vi "UHR-Fleezers Control (host) -Leonardo 04-2018 V3_greenctrl.vi"(0 "Tab Green FB":T5(tab)=enum."Trap Control (RF)") -> ()   [LabVIEW 2013] (continued)
                  n1367 = call "isclickinwindow.vi"("Image Param"=w2127, "Point32"=w2126) -> ("Y px"=w2120:i32, "Height"=w2121:i32, "X px"=w2122:i32, "Width"=w2123:i32, "In image?"=w2125:bool)  [unwired: 1 in]
                  n1368 = Not(x=w2125) -> (.not. x?=w2124:bool)
                }
              }
            }
            n1369 = Not(x=w2078) -> (.not. x?=w2077:bool)
            n1370 = case shown="True" w2077 {
              tunnel: w2075 -> [_ w2141]
              tunnel: w2073 -> [_ w2140]
              tunnel: w2076 -> [_ w2139]
              tunnel: w2074 -> [_ w2138]
              frame False {
              }
              frame True {
                w2134 = FALSE ("Get Point")
                n1371 = local read "Scan lines (y)"() -> (w2143:u64)
                n1372 = local read "Actual MCL Inc (V)"() -> (w2135:dbl)
                n1373 = local read "Scan steps (MCL)"() -> (w2142:u64)
                n1374 = Divide "Y Pix/step"(x=w2138, y=w2143) -> (x/y=w2150:dbl)
                n1375 = Divide "Y V/pix"(x=w2135, y=w2150) -> (x/y=w2149:dbl)
                n1376 = Divide "Y half step offset"(x=w2135, y=2.0) -> (x/y=w2151:dbl)
                n1377 = Divide "X pix/step"(x=w2139, y=w2142) -> (x/y=w2148:dbl)
                n1378 = Negate(x=w2151) -> (-x=w2152:dbl)
                n1379 = local read "Initial Y"() -> (w2158:dbl)
                n1380 = Multiply(x=w2140, y=w2149) -> (x*y=w2159:dbl)
                n1381 = Divide "X half step offset"(x=w2135, y=2.0) -> (x/y=w2145:dbl)
                n1382 = Divide "X V/pix"(x=w2135, y=w2148) -> (x/y=w2147:dbl)
                n1383 = Multiply(x=w2135, y=w2142) -> (x*y=w2154:dbl)
                n1384 = Compound Arithmetic op=ADD(w2152, w2159, w2158) -> (w2136:dbl)
                "Pointer Y (V)" <- w2136
                n1385 = Multiply(x=w2147, y=w2141) -> (x*y=w2156:dbl)
                n1386 = Negate(x=w2145) -> (-x=w2144:dbl)
                n1387 = local read "Initial X"() -> (w2157:dbl)
                n1388 = Negate(x=w2156) -> (-x=w2155:dbl)
                n1389 = Compound Arithmetic op=ADD(w2144, w2154, w2157, w2155) -> (w2137:dbl)
                "Pointer X (V)" <- w2137
                n1390 = Or(x="Set X Only", y="Set Confocal Spot (X-Y)") -> (x .or. y?=w2130:bool)
                n1391 = Or(x="Set Confocal Spot (X-Y)", y="Set Y Only") -> (x .or. y?=w2129:bool)
                n1392 = case shown="True" w2130 {
                  tunnel: w2137 -> [_ w2160]
                  frame False {
                  }
                  frame True {
                    n1393 = property on="AO2" class="Slide (strict)"("Val(Sgnl)"=w2160) -> ()  [unwired: 2 in, 2 out]
                  }
                }
                n1394 = case shown="True" w2129 {
                  tunnel: w2136 -> [_ w2161]
                  frame False {
                  }
                  frame True {
                    n1395 = property on="AO1" class="Slide (strict)"("Val(Sgnl)"=w2161) -> ()  [unwired: 2 in, 2 out]
                  }
                }
                n1396 = local write "Set Confocal Spot (X-Y)"(w2134) -> ()
                n1397 = local write "Set X Only"(w2134) -> ()
                n1398 = local write "Set Y Only"(w2134) -> ()
              }
            }
          }
          frame 3 {
            n1399 = local read "BD 2 Frequency 1 (MHz)"() -> (w2162:dbl)
            n1400 = local read "BD 1 Frequency 1 (MHz)"() -> (w2163:dbl)
            n1401 = local write "Manipulating Trap"(TRUE ("Manipulating Trap")) -> ()
            n1402 = local write "Coords"(T8 {"Horizontal"=0, "Vertical"=0} ("Coords")) -> ()
            n1403 = while {
              tunnel: w2168 -> [w2173]
              tunnel: w2166 -> [w2172]
              tunnel: w2164 -> [w2171]
              tunnel: w2163 -> [w2170]
              tunnel: w2162 -> [w2169]
              stop <- w2174 stop-if-true
              n1404 = event shown="[0] \"Pane\": Mouse Move" {
                selector: _ -> [_ _]
                dyn-events: _ -> [_ _]
                timeout: _ -> [_ _]
                tunnel: ["Force Manip Abort" w2238] -> w2174
                tunnel: w2173 -> [w2181 _]
                tunnel: w2172 -> [w2179 _]
                tunnel: w2171 -> [w2178 _]
                tunnel: w2170 -> [w2177 _]
                tunnel: w2169 -> [w2176 _]
                event Mouse Move {
                  n1405 = event-data() -> ("Time"=w2182:u32, "Coords"=w2183:T8)  [unwired: 3 out]
                  n1406 = Less?(x=w2182, y=w2181) -> (x < y?=w2180:bool)
                  n1407 = case "Makes sure old motion events prior to mouse click aren't used" shown="False" w2180 {
                    tunnel: w2183 -> [w2225 _]
                    tunnel: w2179 -> [w2226 _]
                    tunnel: w2178 -> [w2203 _]
                    tunnel: w2177 -> [w2199 _]
                    tunnel: w2176 -> [w2198 _]
                    frame False {
                      n1408 = Subtract(x=w2225, y=w2226) -> (x-y=w2224:T8)
                      "Coords" <- w2224
                      n1409 = local read "Y RF Frequency Limits (MHz)"() -> (w2184:T16)
                      n1410 = To Double Precision Float(number=w2224) -> (double precision float=w2223:cluster{"Horizontal":dbl, "Vertical":dbl})
                      n1411 = Multiply(x=cluster{"Horizontal":dbl, "Vertical":dbl} {"Horizontal"=-1.0, "Vertical"=1.0}, y="Manipulation Scaling") -> (x*y=w2219:cluster{"Horizontal":dbl, "Vertical":dbl})
                      n1412 = local read "X RF Frequency Limits (MHz)"() -> (w2185:T16)
                      n1413 = Multiply(x=w2223, y=w2219) -> (x*y=w2221:cluster{"Horizontal":dbl, "Vertical":dbl})
                      n1414 = Unbundle By Name(w2221) -> ("Horizontal"=w2216:dbl, "Vertical"=w2220:dbl)
                      n1415 = Unbundle By Name(w2184) -> ("Maximum"=w2187:dbl, "Minimum"=w2186:dbl)
                      n1416 = Boolean To (0,1)(Boolean="Manip. X?") -> (0, 1=w2214:i16)
                      n1417 = Boolean To (0,1)(Boolean="Manip. Y?") -> (0, 1=w2211:i16)
                      n1418 = local read "BD 1 Frequency 2 (MHz)"() -> (w2201:dbl)
                      n1419 = Multiply(x=w2220, y=w2211) -> (x*y=w2213:dbl)
                      n1420 = Multiply(x=w2214, y=w2216) -> (x*y=w2217:dbl)
                      n1421 = local read "BD 2 Frequency 2 (MHz)"() -> (w2200:dbl)
                      n1422 = Unbundle By Name(w2185) -> ("Maximum"=w2189:dbl, "Minimum"=w2188:dbl)
                      n1423 = Add(x=w2198, y=w2213) -> (x+y=w2191:dbl)
                      n1424 = Add(x=w2199, y=w2217) -> (x+y=w2193:dbl)
                      n1425 = In Range and Coerce(upper limit=w2189, x=w2193, lower limit=w2188) -> (coerced(x)=w2192:dbl)  [unwired: 1 out]
                      n1426 = In Range and Coerce(upper limit=w2187, x=w2191, lower limit=w2186) -> (coerced(x)=w2190:dbl)  [unwired: 1 out]
                      n1427 = Subtract(x=w2192, y=w2201) -> (x-y=w2210:dbl)
                      n1428 = Subtract(x=w2190, y=w2200) -> (x-y=w2209:dbl)
                      n1429 = Square(x=w2210) -> (x^2=w2208:dbl)
                      n1430 = Square(x=w2209) -> (x^2=w2207:dbl)
                      n1431 = Add(x=w2208, y=w2207) -> (x+y=w2206:dbl)
                      n1432 = Square Root(x=w2206) -> (sqrt(x)=w2202:dbl)
                      n1433 = In Range and Coerce(upper limit="Limit Max (MHz)", x=w2202, lower limit="Limit Min (MHz)") -> (In Range?=w2195:bool)  [unwired: 1 out]
                      n1434 = Not(x="Limits Enable") -> (.not. x?=w2194:bool)
                      n1435 = Or(x=w2195, y=w2194) -> (x .or. y?=w2196:bool)
                      n1436 = case shown="True" w2196 {
                        tunnel: w2203 -> [_ w2236]
                        tunnel: w2202 -> [_ w2227]
                        tunnel: w2192 -> [_ w2234]
                        tunnel: w2201 -> [_ w2233]
                        tunnel: w2190 -> [_ w2232]
                        tunnel: w2200 -> [_ w2231]
                        tunnel: w2185 -> [_ w2229]
                        tunnel: w2184 -> [_ w2228]
                        frame False {
                        }
                        frame True {
                          n1437 = local read "BD 1 Frequency 3 (MHz)"() -> (w2235:dbl)
                          n1438 = local read "BD 2 Frequency 3 (MHz)"() -> (w2230:dbl)
                          n1439 = local write "Trap Delta (MHz)"(w2227) -> ()
                          n1440 = property on="Initial delta (MHz)" class="DigNum (strict)"("Val(Sgnl)"=w2227) -> ()  [unwired: 2 in, 2 out]
                          n1441 = call "set RF board frequency - interlace.vi"("Board 2 Frequency Limits"=w2228, "Board 1 Frequency Limits"=w2229, "FPGA VI Reference In"=w2236, "Board 2 Frequency 3 (MHz)"=w2230, "Board 1 Frequency 3 (MHz)"=w2235, "Board 2 Frequency 2 (MHz)"=w2231, "Board 2 Frequency 1 (MHz)"=w2232, "Board 1 Frequency 2 (MHz)"=w2233, "Board 1 Frequency 1  (MHz)"=w2234) -> ()  [unwired: 1 in, 2 out]
                          n1442 = local write "BD 2 Frequency 1 (MHz)"(w2232) -> ()
                          n1443 = local write "BD 1 Frequency 1 (MHz)"(w2234) -> ()
                        }
                      }
                    }
                    frame True {
                    }
                  }
                }
                event Mouse Up {
                  n1444 = event-data() -> ("Button"=w2237:u16)  [unwired: 8 out]
                  n1445 = case shown="3" w2237 {
                    tunnel: [FALSE TRUE] -> w2238
                    frame 0, Default {
                    }
                    frame 3 {
                      n1446 = local write "Manipulating Trap"(FALSE ("Manipulating Trap")) -> ()
                    }
                  }
                }
              }
            }
          }
        }
      }
      event Mouse Move {
        n1447 = event-data() -> ()  [unwired: 6 out]
      }
    }
    n1448 = local read "Stop All"() -> (w2059:bool)
    n1449 = node-c288() -> ()  [unwired: 2 out]
  }
  n1450 = node-c288(w53) -> ()  [unwired: 1 out]
  n1451 = node-c288(w102) -> ()  [unwired: 1 out]
  n1452 = node-c288(w109) -> ()  [unwired: 1 out]
  n1453 = node-c288(i64 1 ("Period"), 1 ("Processor")) -> (w195:T25)  [unwired: 2 out]
  n1454 = timed-loop "Acquire Data" {
    tunnel: w61 -> [w2547]
    tunnel: w76 -> [w2546]
    tunnel: [w2577] -> w69
    tunnel: [w2571] -> w2
    timing: w195 -> [_]
    timing-out: [_] -> w194
    tunnel: w93 -> [w2393]
    stop <- "Stop All" stop-if-true
    (unwired) u32 0 ("Number of Elements")
    w2380 = "NI_ChannelName" ("name")
    n1455 = node-c288() -> ()  [unwired: 2 out]
    n1456 = First Call?() -> (First Call?: T/F=w2346:bool)
    n1457 = Or(x="Reset", y=w2346) -> (x .or. y?=w2347:bool)
    n1458 = local read "MCL Tracking"() -> (w2284:bool)
    n1459 = case "Reset data stream" shown="True" w2347 {
      tunnel: w2547 -> [w2697 w2705]
      tunnel: w2546 -> [w2696 w2704]
      tunnel: [w2697 w2699] -> w2282
      tunnel: [w2696 w2698] -> w2542
      frame False {
      }
      frame True {
        w2702 = TRUE ("AI to FIFO")
        n1460 = local write "Overflow (data lost)"(FALSE ("Overflow (data lost)")) -> ()
        n1461 = call "reset FPGA DMA.vi"("error in"=w2704, "FPGA VI Reference In"=w2705) -> ("error out"=w2700:errorcluster, "FPGA VI Reference Out"=w2701:T20)
        n1462 = xnode "Read/Write Control"("FPGA VI Reference In"=w2701, "error in"=w2700, "AI to FIFO"=w2702, "APD to FIFO"=w2702) -> ("FPGA VI Reference Out"=w2699:T20, "error out"=w2698:errorcluster)
      }
    }
    n1463 = Or(x="Start AOD Scan", y="Trap Raster Scan") -> (x .or. y?=w2500:bool)
    n1464 = case "Start AOM raster scan" shown="True" w2500 {
      tunnel: w2282 -> [w3438 w3449]
      tunnel: w2542 -> [w3437 w3448]
      tunnel: [w3438 w3442] -> w2281
      tunnel: [w3437 w3441] -> w2541
      frame False {
      }
      frame True {
        n1465 = case shown="True" "Restart DMA? (AOD)" {
          tunnel: [w3489 w3491] -> w3443
          tunnel: [w3488 w3490] -> w3444
          tunnel: w3449 -> [w3489 w3493]
          tunnel: w3448 -> [w3488 w3492]
          frame False {
          }
          frame True {
            n1466 = local write "Overflow (data lost)"(FALSE ("Overflow (data lost)")) -> ()
            n1467 = call "reset FPGA DMA.vi"("error in"=w3492, "FPGA VI Reference In"=w3493) -> ("error out"=w3490:errorcluster, "FPGA VI Reference Out"=w3491:T20)
          }
        }
        n1468 = local write "Trap Raster Scan"(FALSE ("Trap Raster Scan")) -> ()
        n1469 = case shown="False" "Move MCL Also?" {
          tunnel: w3444 -> [w3453 w3483]
          tunnel: w3443 -> [w3454 w3484]
          tunnel: [w3452 w3487] -> w3442
          tunnel: [w3451 w3486] -> w3441
          tunnel: "Raster to target force?" -> [w3450 w3456]
          frame False {
            w3455 = TRUE ("AI to FIFO")
            n1470 = xnode "Read/Write Control"("FPGA VI Reference In"=w3454, "error in"=w3453, "AI to FIFO"=w3455, "APD to FIFO"=w3455, "Start scan"=w3455, "Raster to target force"=w3450) -> ("FPGA VI Reference Out"=w3452:T20, "error out"=w3451:errorcluster)
          }
          frame True {
            w3480 = FALSE ("1D or 2D Scan?")
            w3485 = TRUE ("AI to FIFO")
            # "Count for MCL loop"
            # "N total cycles"
            # "N steps"
            # "V_int"
            n1471 = local read "Scan Range (nm)"() -> (w3462:dbl)
            n1472 = local read "Number of F/B Scans (AOD)"() -> (w3479:u16)
            n1473 = Sign(1:w3462) -> (0:w3461:dbl)
            n1474 = Compound Arithmetic op=MULTIPLY(w3462, "MCL Step Position Ratio", "MCL/AOM Scale Tweak") -> (w3466:dbl)
            n1475 = Negate(x=w3461) -> (-x=w3458:dbl)
            n1476 = Multiply(x=w3458, y="MCL Step Increment (V_int)") -> (x*y=w3460:dbl)
            n1477 = Divide(x=w3466, y="MCL X Cal (nm/V)") -> (x/y=w3472:dbl)
            n1478 = Multiply(x=32767.0 ("y"), y=w3472) -> (x*y=w3478:dbl)
            n1479 = local read "Total Counts (ticks)"() -> (w3463:u32)
            n1480 = local read "Cycles/step (AOD)"() -> (w3474:u64)
            n1481 = local read "Scan steps (AOD)"() -> (w3475:u64)
            n1482 = Divide(x=w3478, y=10.0) -> (x/y=w3471:dbl)
            n1483 = Divide(x=w3471, y="MCL Step Increment (V_int)") -> (x/y=w3469:dbl)
            n1484 = Absolute Value(x=w3469) -> (abs(x)=w3457:dbl)
            n1485 = Compound Arithmetic op=MULTIPLY(w3475, w3474, w3463) -> (w3470:u64)
            n1486 = local write "wait to reset values"(w3485) -> ()
            n1487 = local write "MCL Scanning"(w3485) -> ()
            n1488 = Divide(x=w3470, y=w3457) -> (x/y=w3467:dbl)
            "MCL Count" <- w3467
            n1489 = xnode "Read/Write Control"("FPGA VI Reference In"=w3484, "error in"=w3483, "Scan steps (MCL)"=w3457, "Number of scans (MCL)"=w3479, "Cycles per step (MCL)"=u64 1, "Scan freq.  increment (MCL)"=w3460, "1D or 2D Scan?"=w3480, "MCL Scan Axis"=w3480, "Cont. Scan (MCL)"=w3480, "MCL count"=w3467) -> ("FPGA VI Reference Out"=w3482:T20, "error out"=w3481:errorcluster)
            n1490 = xnode "Read/Write Control"("FPGA VI Reference In"=w3482, "error in"=w3481, "AI to FIFO"=w3485, "APD to FIFO"=w3485, "Start scan"=w3485, "Start scan (MCL)"=w3485, "Raster to target force"=w3456) -> ("FPGA VI Reference Out"=w3487:T20, "error out"=w3486:errorcluster)
          }
        }
        "Raster Scanning..." <- TRUE ("Scanning...")
      }
    }
    n1491 = And(x="Save scans", y=w2500) -> (x .and. y?=w2540:bool)
    n1492 = Compound Arithmetic op=OR("Start MCL Scan", "Confocal Image", "Confocal Linescan") -> (w2498:bool)
    n1493 = And(x="Save Data (MCL)", y=w2498) -> (x .and. y?=w2539:bool)
    n1494 = case "Start MCL raster scan" shown="True" w2498 {
      tunnel: w2281 -> [w2988 w3003]
      tunnel: w2541 -> [w2987 w3002]
      tunnel: [w2988 w2998] -> w2316
      tunnel: [w2987 w2997] -> w2315
      tunnel: [FALSE w2996] -> w2525
      tunnel: "Start MCL Scan" -> [_ w2991]
      tunnel: "Confocal Image" -> [_ w2990]
      tunnel: "Confocal Linescan" -> [_ _]
      frame False {
      }
      frame True {
        w2996 = TRUE
        n1495 = case shown="True" "Restart DMA? (MCL)" {
          tunnel: [w3048 w3050] -> w3001
          tunnel: [w3047 w3049] -> w3000
          tunnel: w3003 -> [w3048 w3053]
          tunnel: w3002 -> [w3047 w3052]
          frame False {
          }
          frame True {
            n1496 = call "reset FPGA DMA.vi"("error in"=w3052, "FPGA VI Reference In"=w3053) -> ("error out"=w3049:errorcluster, "FPGA VI Reference Out"=w3050:T20)
            n1497 = local write "Overflow (data lost)"(FALSE ("Overflow (data lost)")) -> ()
          }
        }
        n1498 = case shown="False" w2991 {
          selector: w2991 -> [_ w3007]
          tunnel: w2990 -> [w3006 _]
          tunnel: [w3006 w3007] -> w2989
          frame False {
            n1499 = property on="2D or 1D Scan" class="Bool (strict)"("Val(Sgnl)"=w3006) -> ()  [unwired: 2 in, 2 out]
            n1500 = property on="Confocal Image" class="Bool (strict)"("Value"=FALSE ("Start Confocal Map")) -> ()  [unwired: 2 in, 2 out]
          }
          frame True {
          }
        }
        n1501 = local write "MCL Scanning"(w2996) -> ()
        n1502 = local read "AO1"() -> (w2993:dbl)
        n1503 = local read "AO2"() -> (w2992:dbl)
        n1504 = case shown="True" "Center Scan" {
          tunnel: w3001 -> [w3014 w3046]
          tunnel: w3000 -> [w3013 w3045]
          tunnel: [w3012 w3044] -> w2998
          tunnel: [w3011 w3043] -> w2997
          tunnel: [w3009 w3030] -> w2995
          tunnel: [w3008 w3029] -> w2994
          tunnel: w2993 -> [w3009 w3035]
          tunnel: w2992 -> [w3008 w3038]
          tunnel: w2989 -> [_ _]
          frame False {
            w3010 = TRUE ("AI to FIFO")
            n1505 = xnode "Read/Write Control"("FPGA VI Reference In"=w3014, "error in"=w3013, "AI to FIFO"=w3010, "APD to FIFO"=w3010, "Start scan (MCL)"=w3010) -> ("FPGA VI Reference Out"=w3012:T20, "error out"=w3011:errorcluster)
          }
          frame True {
            w3042 = TRUE ("AI to FIFO")
            n1506 = local read "Scan steps (MCL)"() -> (w3021:u64)
            n1507 = local read "Scan lines (y)"() -> (w3017:u64)
            n1508 = local read "Fast Scan Dir"() -> (w3028:bool)
            n1509 = local read "Actual MCL Inc (V)"() -> (w3018:dbl)
            n1510 = Decrement(x=w3017) -> (x-1=w3016:u64)
            n1511 = Decrement(x=w3021) -> (x-1=w3020:u64)
            n1512 = Multiply(x=w3018, y=w3016) -> (x*y=w3015:dbl)
            n1513 = Divide(x=w3015, y=2.0) -> (x/y=w3025:dbl)
            n1514 = Multiply(x=w3018, y=w3020) -> (x*y=w3019:dbl)
            n1515 = Divide(x=w3019, y=2.0) -> (x/y=w3024:dbl)
            n1516 = Select(t=w3024, s=w3028, f=w3025) -> (s? t:f=w3023:dbl)
            n1517 = Select(t=w3025, s=w3028, f=w3024) -> (s? t:f=w3027:dbl)
            n1518 = Subtract(x=w3035, y=w3027) -> (x-y=w3026:dbl)
            n1519 = Subtract(x=w3038, y=w3023) -> (x-y=w3022:dbl)
            n1520 = local read "2D or 1D Scan"() -> (w3040:bool)
            n1521 = Not(x=w3028) -> (.not. x?=w3034:bool)
            n1522 = Not(x=w3040) -> (.not. x?=w3036:bool)
            n1523 = And(x=w3028, y=w3036) -> (x .and. y?=w3037:bool)
            n1524 = And(x=w3036, y=w3034) -> (x .and. y?=w3039:bool)
            n1525 = Select(t=w3038, s=w3039, f=w3022) -> (s? t:f=w3029:dbl)
            n1526 = Select(t=w3035, s=w3037, f=w3026) -> (s? t:f=w3030:dbl)
            n1527 = call "Volt to I16.vi"("Voltage In"=w3030) -> ("I16 Voltage Out"=w3033:i16)
            n1528 = call "Volt to I16.vi"("Voltage In"=w3029) -> ("I16 Voltage Out"=w3032:i16)
            n1529 = xnode "Read/Write Control"("FPGA VI Reference In"=w3046, "error in"=w3045, "AI to FIFO"=w3042, "APD to FIFO"=w3042, "Start scan (MCL)"=w3042, "AO1 (Y)"=w3033, "AO2 (X)"=w3032) -> ("FPGA VI Reference Out"=w3044:T20, "error out"=w3043:errorcluster)
          }
        }
        "Initial Y" <- w2995
        "Initial X" <- w2994
        "wait to reset values" <- w2996
      }
    }
    n1530 = local read "Trap Pos Elements/DMA read"() -> (w2389:u32)
    n1531 = local read "Trap AI Elements/DMA read"() -> (w2314:u32)
    n1532 = local read "APD Elements/DMA read"() -> (w2428:u32)
    n1533 = local read "Trap AI FIFO Depth"() -> (w2587:u32)
    n1534 = xnode "Invoke Method"("FPGA VI Reference In"=w2316, "error in"=w2315, "Number of Elements"=w2389, "Timeout (ms)"=-1) -> ("Data"=w2353:u16[], "Elements Remaining"=→"Trap Pos FIFO El Remaining":u32)  [unwired: 2 out]
    n1535 = xnode "Invoke Method"("FPGA VI Reference In"=w2316, "error in"=w2315, "Number of Elements"=w2314, "Timeout (ms)"=-1 ("Timeout")) -> ("FPGA VI Reference Out"=w2285:T20, "error out"=w2317:errorcluster, "Data"=w2313:i16[], "Elements Remaining"=w2318:u32)
    "Trap AI FIFO El. Rem." <- w2318
    n1536 = xnode "Get APD Data"("FPGA VI Reference In"=w2316, "error in"=w2315, "Number of Elements"=w2428, "Timeout (ms)"=-1) -> ("Data"=w2427:u32[], "Elements Remaining"=→"APD FIFO Elements Remaining":u32)  [unwired: 2 out]
    n1537 = Subtract(x=w2587, y=w2314) -> (x-y=w2586:u32)
    n1538 = Decimate 1D Array(w2353) -> (w2350:u16[], w2352:u16[], w2351:u16[])
    n1539 = Divide(x=w2318, y=w2586) -> (x/y=w2585:dbl)
    "Buffer Status" <- w2585
    n1540 = To Unsigned Long Integer(number=w2350) -> (unsigned 32bit integer=w2349:u32[])
    n1541 = Join Numbers(hi=w2352, lo=w2351) -> ((hi.lo)=w2348:u32[])
    n1542 = Equal?(x=w2585, y=1.0) -> (x = y?=w2583:bool)
    n1543 = Join Numbers(hi=w2349, lo=w2348) -> ((hi.lo)=w2342:u64[])
    n1544 = call "IR AOM word to freq - vec.vi"("Frequency Word In (double vec)"=w2342) -> ("Frequency Out"=w2388:dbl[])
    n1545 = case "Alert buffer overflow" shown="True" w2583 {
      frame False {
      }
      frame True {
        n1546 = call <vilib>:"Beep.vi"() -> ()  [unwired: 3 in, 9 out]
        "Overflow (data lost)" <- TRUE ("Overflow (data lost)")
      }
    }
    n1547 = Decimate 1D Array(w2388) -> (w2387:dbl[], w2386:dbl[])
    n1548 = Array Size(array=w2313) -> (size(s)=→"Waveform Chart":i32)
    n1549 = Build Array(w2387, w2386) -> (w2385:dbl[][])
    n1550 = local read "Trap Sets"() -> (w2460:u32)
    n1551 = case "Deinterlace trap data, average down PSD" shown="2" w2460 {
      tunnel: w2313 -> [w3083 w3148]
      tunnel: [w3080 w3145] -> w2453
      tunnel: [w3083 w3147] -> w2345
      tunnel: "Detector Type" -> [w3082 w3143]
      tunnel: [w3081 w3146] -> w2452
      tunnel: [w3079 w3144] -> w2558
      frame 1, Default {
        n1552 = Divide(x=w3083, y=3276.7) -> (x/y=w3084:dbl[])
        n1553 = Decimate 1D Array(w3084) -> (w3093:dbl[], w3092:dbl[], w3091:dbl[], w3090:dbl[], w3089:dbl[], w3088:dbl[], w3087:dbl[], w3086:dbl[])
        n1554 = case shown="\"IR-QPD + PSD + FB-QPD position\"" w3082 {
          tunnel: w3093 -> [w3117 w3142]
          tunnel: w3092 -> [w3116 w3141]
          tunnel: w3091 -> [w3101 w3119]
          tunnel: w3090 -> [w3102 w3129]
          tunnel: w3089 -> [w3115 w3140]
          tunnel: w3088 -> [w3114 w3139]
          tunnel: w3087 -> [w3098 w3120]
          tunnel: w3086 -> [w3097 w3118]
          tunnel: [w3096 w3126] -> w3081
          tunnel: [w3095 w3125] -> w3080
          tunnel: [w3094 w3124] -> w3079
          frame "IR-QPD + PSD + FB-QPD", Default {
            w3094 = 0  # Channel pattern
            n1555 = Divide(x=w3117, y=w3102) -> (x/y=w3104:dbl[])
            n1556 = Divide(x=w3116, y=w3102) -> (x/y=w3103:dbl[])
            n1557 = Divide(x=w3115, y=w3098) -> (x/y=w3100:dbl[])
            n1558 = Divide(x=w3114, y=w3097) -> (x/y=w3099:dbl[])
            n1559 = Build Array(w3104, w3103, w3102, w3101, w3100, w3099, w3098, w3097) -> (w3095:dbl[][])
            n1560 = Bundle("T1 Y", "T1 X", "T1 Sum", "FB Sum", "PSD Y", "PSD X", "PSD Y Sum", "PSD X Sum") -> (w3113:T42)  [unwired: 1 out]
            n1561 = Cluster To Array(cluster=w3113) -> (array=w3096:string[])
          }
          frame "IR-QPD + PSD + FB-QPD position" {
            w3124 = 3  # Channel pattern
            n1562 = Negate(x=w3120) -> (-x=w3121:dbl[])
            n1563 = Divide(x=w3142, y=w3129) -> (x/y=w3131:dbl[])
            n1564 = Divide(x=w3141, y=w3129) -> (x/y=w3130:dbl[])
            n1565 = Divide(x=w3140, y=w3120) -> (x/y=w3128:dbl[])
            n1566 = Divide(x=w3139, y=w3121) -> (x/y=w3127:dbl[])
            n1567 = Build Array(w3131, w3130, w3129, w3118, w3119, w3128, w3127, w3120) -> (w3125:dbl[][])
            n1568 = Bundle("T1 Y", "T1 X", "T1 Sum", "FB X", "FB Sum", "PSD Y", "PSD X", "PSD Y Sum") -> (w3138:T42)  [unwired: 1 out]
            n1569 = Cluster To Array(cluster=w3138) -> (array=w3126:string[])
          }
        }
      }
      frame 2 {
        n1570 = case shown="\"UCB Fleezers 052511\"" w3143 {
          tunnel: w3148 -> [w3210 w3277 w3316 w3416]
          tunnel: [w3149 w3269 w3312 w3347] -> w3147
          tunnel: [w3176 w3260 w3314 w3394] -> w3146
          tunnel: [w3175 w3224 w3305 w3361] -> w3145
          tunnel: [w3169 w3259 w3346 w3392] -> w3144
          frame "IR-QPD + PSD + FB-QPD", Default {
            w3169 = 1  # Channel pattern
            # "time average x2 the 4th signal and the 4 psd signals (detection laser)"
            # "deinterlace 3 signals from qpd"
            n1571 = Decimate 1D Array(w3210) -> (w3209:i16[], w3208:i16[], w3174:i16[], w3207:i16[], w3197:i16[], w3195:i16[], w3194:i16[], w3192:i16[])
            n1572 = call "downsample 1D array - double.vi"("Ave N"=2.0, "Array In"=w3197) -> ("Array Out"=w3196:dbl[])  [unwired: 1 out]
            n1573 = call "downsample 1D array - double.vi"("Ave N"=2.0, "Array In"=w3192) -> ("Array Out"=w3191:dbl[])  [unwired: 1 out]
            n1574 = call "downsample 1D array - double.vi"("Ave N"=2.0, "Array In"=w3194) -> ("Array Out"=w3193:dbl[])  [unwired: 1 out]
            n1575 = call "downsample 1D array - double.vi"("Ave N"=2.0, "Array In"=w3195) -> ("Array Out"=w3177:dbl[])  [unwired: 1 out]
            n1576 = Decimate 1D Array(w3209) -> (w3206:i16[], w3178:i16[])
            n1577 = Decimate 1D Array(w3208) -> (w3205:i16[], w3203:i16[])
            n1578 = Decimate 1D Array(w3207) -> (w3204:i16[], w3202:i16[])
            n1579 = Decimate 1D Array(w3174) -> (w3173:i16[], w3172:i16[])
            n1580 = Interleave 1D Arrays(w3206, w3205, w3204, w3178, w3203, w3202, w3173, w3172, w3196, w3177, w3193, w3191) -> (w3190:dbl[])
            n1581 = To Word Integer(number=w3190) -> (16bit integer=w3149:i16[])
            n1582 = Divide(x=w3190, y=3276.7) -> (x/y=w3189:dbl[])
            n1583 = Decimate 1D Array(w3189) -> (w3188:dbl[], w3187:dbl[], w3186:dbl[], w3185:dbl[], w3184:dbl[], w3183:dbl[], w3171:dbl[], w3170:dbl[], w3182:dbl[], w3181:dbl[], w3180:dbl[], w3179:dbl[])
            n1584 = Divide(x=w3188, y=w3186) -> (x/y=w3156:dbl[])
            n1585 = Divide(x=w3187, y=w3186) -> (x/y=w3155:dbl[])
            n1586 = Divide(x=w3185, y=w3183) -> (x/y=w3154:dbl[])
            n1587 = Divide(x=w3184, y=w3183) -> (x/y=w3153:dbl[])
            n1588 = Divide(x=w3182, y=w3180) -> (x/y=w3152:dbl[])
            n1589 = Divide(x=w3181, y=w3179) -> (x/y=w3151:dbl[])
            n1590 = Bundle("T1 Y", "T1 X", "T1 Sum", "T2 Y", "T2 X", "T2 Sum", "T1 FB Sum", "T2 FB Sum", "PSD Y", "PSD X", "PSD Y Sum", "PSD X Sum") -> (w3157:T43)  [unwired: 1 out]
            n1591 = Build Array(w3156, w3155, w3186, w3154, w3153, w3183, w3171, w3170, w3152, w3151, w3180, w3179) -> (w3175:dbl[][])
            n1592 = Cluster To Array(cluster=w3157) -> (array=w3176:string[])
          }
          frame "IR-QPD + PSD + FB-QPD X position" {
            w3259 = 2  # Channel pattern
            # "convert\nADC numbers\nto volts"
            # "time average x2 the 3 psd signals (detection laser)"
            # "deinterlace 3 signals from qpds"
            n1593 = Decimate 1D Array(w3277) -> (w3276:i16[], w3275:i16[], w3212:i16[], w3213:i16[], w3222:i16[], w3219:i16[], w3216:i16[], w3247:i16[])
            n1594 = Decimate 1D Array(w3276) -> (w3274:i16[], w3261:i16[])
            n1595 = call "downsample 1D array - I16.vi"("Ave N"=2.0, "Array In"=w3222) -> ("Array Out"=w3220:i16[])  [unwired: 1 in]
            n1596 = call "downsample 1D array - I16.vi"("Ave N"=2.0, "Array In"=w3219) -> ("Array Out"=w3217:i16[])  [unwired: 1 in]
            n1597 = Decimate 1D Array(w3275) -> (w3273:i16[], w3271:i16[])
            n1598 = Decimate 1D Array(w3213) -> (w3272:i16[], w3270:i16[])
            n1599 = Decimate 1D Array(w3247) -> (w3246:i16[], w3244:i16[])
            n1600 = Decimate 1D Array(w3212) -> (w3245:i16[], w3243:i16[])
            n1601 = call "downsample 1D array - I16.vi"("Ave N"=2.0, "Array In"=w3216) -> ("Array Out"=w3214:i16[])  [unwired: 1 in]
            n1602 = Interleave 1D Arrays(w3274, w3273, w3272, w3261, w3271, w3270, w3246, w3245, w3244, w3243, w3220, w3217, w3214) -> (w3269:i16[])
            n1603 = Divide(x=w3269, y=3276.7) -> (x/y=w3268:dbl[])
            n1604 = Decimate 1D Array(w3268) -> (w3267:dbl[], w3266:dbl[], w3265:dbl[], w3264:dbl[], w3263:dbl[], w3262:dbl[], w3235:dbl[], w3233:dbl[], w3232:dbl[], w3230:dbl[], w3229:dbl[], w3228:dbl[], w3225:dbl[])
            n1605 = Divide(x=w3267, y=w3265) -> (x/y=w3251:dbl[])
            n1606 = Divide(x=w3266, y=w3265) -> (x/y=w3250:dbl[])
            n1607 = Divide(x=w3264, y=w3262) -> (x/y=w3249:dbl[])
            n1608 = Divide(x=w3263, y=w3262) -> (x/y=w3248:dbl[])
            n1609 = Divide(x=w3235, y=w3233) -> (x/y=w3234:dbl[])
            n1610 = Divide(x=w3232, y=w3230) -> (x/y=w3231:dbl[])
            n1611 = Divide(x=w3229, y=w3225) -> (x/y=w3227:dbl[])
            n1612 = Negate(x=w3225) -> (-x=w3223:dbl[])
            n1613 = Divide(x=w3228, y=w3223) -> (x/y=w3226:dbl[])
            n1614 = Bundle("T1 Y", "T1 X", "T1 Sum", "T2 Y", "T2 X", "T2 Sum", "T1 FB X", "T1 FB Sum", "T2 FB X", "T2 FB Sum", "PSD Y", "PSD X", "PSD Y Sum") -> (w3252:T44)  [unwired: 1 out]
            n1615 = Build Array(w3251, w3250, w3265, w3249, w3248, w3262, w3234, w3233, w3231, w3230, w3227, w3226, w3225) -> (w3224:dbl[][])
            n1616 = Cluster To Array(cluster=w3252) -> (array=w3260:string[])
          }
          frame "UCB Fleezers 052511" {
            w3346 = 2  # Channel pattern
            n1617 = Select(t=i16 -1, s="Negate X signals", f=i16 1) -> (s? t:f=w3286:i16)
            n1618 = Decimate 1D Array(w3316) -> (w3287:i16[], w3288:i16[], w3299:i16[], w3315:i16[], w3284:i16[], w3282:i16[], w3280:i16[], w3296:i16[])
            n1619 = Multiply(x=w3286, y=w3288) -> (x*y=w3285:i16[])
            n1620 = Decimate 1D Array(w3287) -> (w3344:i16[], w3334:i16[])
            n1621 = Decimate 1D Array(w3285) -> (w3343:i16[], w3342:i16[])
            n1622 = Decimate 1D Array(w3299) -> (w3293:i16[], w3292:i16[])
            n1623 = Decimate 1D Array(w3315) -> (w3298:i16[], w3297:i16[])
            n1624 = Decimate 1D Array(w3282) -> (w3281:i16[])  [unwired: 1 out]
            n1625 = Decimate 1D Array(w3296) -> (w3295:i16[], w3294:i16[])
            n1626 = Decimate 1D Array(w3280) -> (w3279:i16[])  [unwired: 1 out]
            n1627 = Decimate 1D Array(w3284) -> (w3283:i16[])  [unwired: 1 out]
            n1628 = Interleave 1D Arrays(w3344, w3343, w3298, w3334, w3342, w3297, w3295, w3293, w3294, w3292, w3283, w3281, w3279) -> (w3312:i16[])
            n1629 = Divide(x=w3312, y=3276.7) -> (x/y=w3341:dbl[])
            n1630 = Decimate 1D Array(w3341) -> (w3340:dbl[], w3339:dbl[], w3338:dbl[], w3337:dbl[], w3336:dbl[], w3335:dbl[], w3311:dbl[], w3309:dbl[], w3308:dbl[], w3306:dbl[], w3304:dbl[], w3301:dbl[], w3302:dbl[])
            n1631 = Divide(x=w3340, y=w3338) -> (x/y=w3321:dbl[])
            n1632 = Divide(x=w3339, y=w3338) -> (x/y=w3320:dbl[])
            n1633 = Divide(x=w3337, y=w3335) -> (x/y=w3319:dbl[])
            n1634 = Divide(x=w3336, y=w3335) -> (x/y=w3318:dbl[])
            n1635 = Divide(x=w3311, y=w3309) -> (x/y=w3310:dbl[])
            n1636 = Divide(x=w3308, y=w3306) -> (x/y=w3307:dbl[])
            n1637 = Divide(x=w3304, y=w3302) -> (x/y=w3303:dbl[])
            n1638 = Divide(x=w3301, y=w3302) -> (x/y=w3300:dbl[])
            n1639 = Build Array(w3321, w3320, w3338, w3319, w3318, w3335, w3310, w3309, w3307, w3306, w3303, w3300, w3302) -> (w3305:dbl[][])
            n1640 = Bundle("T1 Y", "T1 X", "T1 Sum", "T2 Y", "T2 X", "T2 Sum", "T1 FB X", "T2 FB Sum", "T2 FB X", "T2 FB Sum", "PSD Y", "PSD X", "PSD Sum") -> (w3322:T44)  [unwired: 1 out]
            n1641 = Cluster To Array(cluster=w3322) -> (array=w3314:string[])
          }
          frame "IR-QPD + PSD + FB-QPD XY positions" {
            w3392 = 4  # Channel pattern
            # "time average x2 the 3 psd signals (detection laser)"
            # "deinterlace 3 signals from qpds"
            n1642 = Decimate 1D Array(w3416) -> (w3415:i16[], w3414:i16[], w3393:i16[], w3413:i16[], w3359:i16[], w3405:i16[], w3404:i16[], w3381:i16[])
            n1643 = Decimate 1D Array "QPD Y"(w3415) -> (w3412:i16[], w3395:i16[])
            n1644 = call "downsample 1D array - double.vi"("Ave N"=2.0, "Array In"=w3405) -> ("Array Out"=w3380:dbl[])  [unwired: 1 out]
            n1645 = call "downsample 1D array - double.vi"("Ave N"=2.0, "Array In"=w3404) -> ("Array Out"=w3379:dbl[])  [unwired: 1 out]
            n1646 = Decimate 1D Array "Feedback Sum"(w3393) -> (w3377:i16[], w3375:i16[])
            n1647 = Decimate 1D Array "Feedback Y"(w3359) -> (w3358:i16[], w3357:i16[])
            n1648 = Decimate 1D Array "Feedback X"(w3381) -> (w3378:i16[], w3376:i16[])
            n1649 = Decimate 1D Array "QPD Sum"(w3413) -> (w3410:i16[], w3408:i16[])
            n1650 = Decimate 1D Array "QPD X"(w3414) -> (w3411:i16[], w3409:i16[])
            n1651 = Interleave 1D Arrays(w3412, w3411, w3410, w3395, w3409, w3408, w3358, w3378, w3377, w3357, w3376, w3375, w3380, w3379) -> (w3403:dbl[])
            n1652 = To Word Integer(number=w3403) -> (16bit integer=w3347:i16[])
            n1653 = Divide(x=w3403, y=3276.7) -> (x/y=w3402:dbl[])
            n1654 = Decimate 1D Array(w3402) -> (w3401:dbl[], w3400:dbl[], w3399:dbl[], w3398:dbl[], w3397:dbl[], w3396:dbl[], w3354:dbl[], w3368:dbl[], w3352:dbl[], w3353:dbl[], w3366:dbl[], w3350:dbl[], w3364:dbl[], w3362:dbl[])
            n1655 = Divide(x=w3401, y=w3399) -> (x/y=w3385:dbl[])
            n1656 = Divide(x=w3400, y=w3399) -> (x/y=w3384:dbl[])
            n1657 = Divide(x=w3398, y=w3396) -> (x/y=w3383:dbl[])
            n1658 = Divide(x=w3397, y=w3396) -> (x/y=w3382:dbl[])
            n1659 = Divide(x=w3354, y=w3352) -> (x/y=w3351:dbl[])
            n1660 = Divide(x=w3368, y=w3352) -> (x/y=w3367:dbl[])
            n1661 = Divide(x=w3353, y=w3350) -> (x/y=w3349:dbl[])
            n1662 = Divide(x=w3366, y=w3350) -> (x/y=w3365:dbl[])
            n1663 = Negate(x=w3362) -> (-x=w3360:dbl[])
            n1664 = Divide(x=w3364, y=w3360) -> (x/y=w3363:dbl[])
            n1665 = Bundle("T1 Y", "T1 X", "T1 Sum", "T2 Y", "T2 X", "T2 Sum", "T1 FB Y", "T1 FB X", "T1 FB Sum", "T2 FB Y", "T2 FB X", "T2 FB Sum", "PSD X", "PSD Y Sum") -> (w3348:T45)  [unwired: 1 out]
            n1666 = Build Array(w3385, w3384, w3399, w3383, w3382, w3396, w3351, w3367, w3352, w3349, w3365, w3350, w3363, w3362) -> (w3361:dbl[][])
            n1667 = Cluster To Array(cluster=w3348) -> (array=w3394:string[])
          }
        }
      }
    }
    "AI labels" <- w2452
    n1668 = xnode "Read/Write Control"("FPGA VI Reference In"=w2285) -> ("FPGA VI Reference Out"=w2278:T20, "BD1 Frequency Out 1"=w2299:u64)  [unwired: 1 in, 1 out]
    n1669 = local read "BD 1 Frequency 2 (MHz)"() -> (w2290:dbl)
    n1670 = To Double Precision Float(number=w2299) -> (double precision float=w2296:dbl)
    n1671 = Multiply(x=49125000.0, y=6.0) -> (x*y=w2295:dbl)
    n1672 = Multiply(x=w2296, y=w2295) -> (x*y=w2293:dbl)
    n1673 = Scale By Power Of 2(n=-48, x=w2293) -> (x*2^n=w2292:dbl)
    n1674 = local read "Dynamic Force FB"() -> (w2289:bool)
    n1675 = local read "Trap Pos. FB ON"() -> (w2288:bool)
    n1676 = Divide(x=w2292, y=1000000.0) -> (x/y=w2283:dbl)
    n1677 = case shown="True" w2284 {
      tunnel: w2283 -> [_ w2674]
      tunnel: w2281 -> [_ w2661]
      frame False {
      }
      frame True {
        n1678 = local read "AOM X Cal (nm/MHz)"() -> (w2671:dbl)
        n1679 = local read "Zero T1 position"() -> (w2673:dbl)
        n1680 = Subtract(x=w2674, y=w2673) -> (x-y=w2672:dbl)
        n1681 = Multiply(x=w2672, y=w2671) -> (x*y=w2670:dbl)
        n1682 = local read "MCL X Cal (nm/V)"() -> (w2667:dbl)
        n1683 = Multiply(x=w2670, y="Tracking factor") -> (x*y=w2668:dbl)
        n1684 = local read "Zero MCL x position"() -> (w2666:dbl)
        n1685 = Divide(x=w2668, y=w2667) -> (x/y=w2665:dbl)
        n1686 = Add(x=w2666, y=w2665) -> (x+y=w2658:dbl)
        "Current MCL (V)" <- w2658
        n1687 = Multiply(x=w2658, y=32767.0) -> (x*y=w2662:dbl)
        n1688 = Divide(x=w2662, y=10.0) -> (x/y=w2659:dbl)
        n1689 = To Word Integer(number=w2659) -> (16bit integer=w2660:i16)
        n1690 = xnode "Read/Write Control"("FPGA VI Reference In"=w2661, "AO2 (X)"=w2660) -> ()  [unwired: 1 in, 2 out]
      }
    }
    n1691 = Subtract(x=w2290, y=w2283) -> (x-y=w2279:dbl)
    "Current deltaFreq" <- w2279
    n1692 = Compound Arithmetic op=AND(w2289, w2288, "Real time offset \ncorrection for setpoint") -> (w2286:bool)
    n1693 = case shown="True" w2286 {
      tunnel: w2279 -> [_ w2677]
      tunnel: w2278 -> [_ w2676]
      frame False {
      }
      frame True {
        n1694 = local read "T1 kappa_x (pN/nm)"() -> (w2685:dbl)
        n1695 = local read "T1 alpha_x (nm/V)"() -> (w2686:dbl)
        n1696 = local read "Negate offset difference"() -> (w2687:bool)
        n1697 = local read "Offset file step size"() -> (w2695:dbl)
        n1698 = Multiply(x="Target Force (pN)", y=2.0) -> (x*y=w2683:dbl)
        n1699 = local read "Setpoint offset\nCorrection values"() -> (w2692:dbl[])
        n1700 = Divide(x=w2677, y=w2695) -> (x/y=w2694:dbl)
        n1701 = Select(t=-1, s=w2687, f=1) -> (s? t:f=w2688:i32)
        n1702 = To Long Integer(number=w2694) -> (32bit integer=w2693:i32)
        n1703 = Multiply(x=w2686, y=w2685) -> (x*y=w2682:dbl)
        n1704 = Divide(x=w2683, y=w2682) -> (x/y=w2681:dbl)
        n1705 = Index Array(array=w2692, index=w2693) -> (element=w2691:dbl)
        n1706 = Multiply(x=w2688, y=w2691) -> (x*y=w2680:dbl)
        n1707 = Add(x=w2681, y=w2680) -> (x+y=w2679:dbl)
        n1708 = To Fixed-Point(number=w2679) -> (fixed-point=w2675:fxp<+/-,16,1>)  [unwired: 1 in]
        "Actual setpoint" <- w2675
        n1709 = xnode "Read/Write Control"("FPGA VI Reference In"=w2676, "Trap Pos. FB SP"=w2675) -> ()  [unwired: 1 in, 2 out]
      }
    }
    n1710 = case shown="True" "Take full offset\n data for display" {
      tunnel: [w2644 w2650] -> w2477
      tunnel: [w2643 w2649] -> w2475
      tunnel: w2279 -> [_ w2656]
      frame False {
        n1711 = Divide(x="T2 offset_x (mV)", y=1000.0) -> (x/y=w2643:dbl)
        n1712 = Divide(x="T1 offset_x (mV)", y=1000.0) -> (x/y=w2644:dbl)
      }
      frame True {
        n1713 = local read "Offset Values"() -> (w2657:T14)
        n1714 = local read "Offset file step size"() -> (w2655:dbl)
        n1715 = Unbundle By Name(w2657) -> ("Trap 1X offset"=w2652:dbl[], "Trap 2X offset"=w2651:dbl[])
        n1716 = Divide(x=w2656, y=w2655) -> (x/y=w2654:dbl)
        n1717 = To Long Integer(number=w2654) -> (32bit integer=w2653:i32)
        n1718 = Index Array(array=w2652, index=w2653) -> (element=w2650:dbl)
        n1719 = Index Array(array=w2651, index=w2653) -> (element=w2649:dbl)
      }
    }
    n1720 = Decimate 1D Array(w2427) -> (w2450:u32[], w2395:u32[])
    n1721 = local read "DMA Update Period (s)"() -> (w2461:dbl)
    n1722 = local read "BD 1 Frequency 2 (MHz)"() -> (w2337:dbl)
    n1723 = local read "BD 1 Frequency 1 (MHz)"() -> (w2338:dbl)
    n1724 = Build Array(w2450, w2395) -> (w2522:u32[][])
    n1725 = local read "Data Period (s)"() -> (w2440:dbl)
    n1726 = Decimate 1D Array(w2345) -> (w2368:i16[], w2367:i16[], w2365:i16[], w2364:i16[])  [unwired: 9 out]
    n1727 = To Double Precision Float(number=w2522) -> (double precision float=w2523:dbl[][])
    n1728 = local read "APD Integration Time (s)"() -> (w2408:dbl)
    n1729 = Divide(x=w2368, y=w2367) -> (x/y=w2369:dbl[])
    n1730 = Divide(x=w2365, y=w2364) -> (x/y=w2366:dbl[])
    n1731 = feedback #1(0.0) -> (w2382:dbl)
    n1732 = Add(x=w2461, y=w2382) -> (x+y=w2560:dbl)
    n1733 = feedback-in #1(w2560) -> ()
    n1734 = local read "AOM X Cal (nm/MHz)"() -> (w2335:dbl)
    n1735 = To Time Stamp(1:w2382) -> (0:w2381:timestamp)
    n1736 = Split 1D Array(array=w2369, index="N El. to Ave.") -> (second subarray=w2372:dbl[])  [unwired: 1 out]
    n1737 = Split 1D Array(array=w2366, index="N El. to Ave.") -> (second subarray=w2371:dbl[])  [unwired: 1 out]
    n1738 = local read "Trap X AI1 (DMA)"() -> (w2370:T13)
    n1739 = Multiply(x=w2440, y="Trap Disp. Downsample") -> (x*y=w2383:dbl)
    "Display Period (s)" <- w2383
    n1740 = Bundle("BD 1 Frequency 1 (MHz)"=w2338, "BD 1 Frequency 2 (MHz)"=w2337) -> (w2339:T46)  [unwired: 1 out]
    n1741 = for "Trap AI" {
      tunnel: [w3078] -> w2554 mode=indexing
      tunnel: w2381 -> [w3068]
      tunnel: "Trap Disp. Downsample" -> [w3076]
      tunnel: w2453 -> [w3074] mode=indexing
      tunnel: w2440 -> [w3073]
      tunnel: w2452 -> [w3072] mode=indexing
      tunnel: w2380 -> [w3071]
      tunnel: [w3070] -> w2419 mode=indexing
      tunnel: w2383 -> [w3069]
      n1742 = Bundle By Name("Y"=w3074, "dt"=w3073) -> (w3075:waveform(dbl))  [unwired: 1 out]
      n1743 = Set Waveform Attribute(5:w3072, 6:w3071, 7:w3075) -> (3:w3070:waveform(dbl))  [unwired: 1 in, 2 out]
      n1744 = call "downsample 1D array - double.vi"("Ave N"=w3076, "Array In"=w3074) -> ("Array Out"=w3077:dbl[])  [unwired: 1 out]
      n1745 = Bundle By Name(cluster=w3070, "t0"=w3068, "Y"=w3077, "dt"=w3069) -> (w3078:waveform(dbl))
    }
    n1746 = call-poly <vilib>:"Mean.vi"("X"=w2371) -> ("mean"=w2359:dbl)  [unwired: 1 out]
    n1747 = call-poly <vilib>:"Mean.vi"("X"=w2372) -> ("mean"=w2360:dbl)  [unwired: 1 out]
    n1748 = Cluster To Array(cluster=w2339) -> (array=w2336:dbl[])
    n1749 = Reciprocal(x=w2383) -> (1/x=→"Trap Disp. Freq. (Hz)":dbl)
    n1750 = local read "Data points/scans (MCL)"() -> (w2534:dbl)
    n1751 = To Fixed-Point(number=w2359) -> (fixed-point=w2357:fxp<+/-,16,1>)  [unwired: 1 in]
    n1752 = To Fixed-Point(number=w2360) -> (fixed-point=w2358:fxp<+/-,16,1>)  [unwired: 1 in]
    n1753 = Bundle("Trap 1 Pos.", "Trap 2 Pos.") -> (w2379:cluster{string, string})  [unwired: 1 out]
    n1754 = Bundle By Name(cluster=w2370, "Set 1"=w2358, "Set 2"=w2357) -> (→"Trap X AI1 (DMA)":T13)
    n1755 = Cluster To Array(cluster=w2379) -> (array=w2376:string[])
    n1756 = for "Trap Position" {
      tunnel: w2385 -> [w2718] mode=indexing
      tunnel: "Trap Disp. Downsample" -> [w2717]
      tunnel: w2383 -> [w2715]
      tunnel: w2381 -> [w2714]
      tunnel: w2380 -> [w2712]
      tunnel: w2376 -> [w2711] mode=indexing
      tunnel: [w2710] -> w2334 mode=indexing
      tunnel: w2336 -> [w2708] mode=indexing
      tunnel: w2335 -> [w2706]
      n1757 = call "downsample 1D array - double.vi"("Ave N"=w2717, "Array In"=w2718) -> ("Array Out"=w2716:dbl[])  [unwired: 1 out]
      n1758 = Subtract(x=w2716, y=w2708) -> (x-y=w2709:dbl[])
      n1759 = Multiply(x=w2706, y=w2709) -> (x*y=w2707:dbl[])
      n1760 = Bundle By Name("Y"=w2707, "dt"=w2715, "t0"=w2714) -> (w2713:waveform(dbl))  [unwired: 1 out]
      n1761 = Set Waveform Attribute(5:w2711, 6:w2712, 7:w2713) -> (3:w2710:waveform(dbl))  [unwired: 1 in, 2 out]
    }
    "Trap Positions" <- w2334
    n1762 = Bundle("APD 1", "APD 2") -> (w2553:cluster{string, string})  [unwired: 1 out]
    n1763 = Cluster To Array(cluster=w2553) -> (array=w2550:string[])
    n1764 = for "APD" {
      tunnel: w2523 -> [w3057] mode=indexing
      tunnel: w2408 -> [w3065]
      tunnel: [w3061] -> w2415 mode=indexing
      tunnel: "APD Disp. Scale" -> [w3062]
      tunnel: w2380 -> [w3060]
      tunnel: w2550 -> [w3059] mode=indexing
      tunnel: "APD Disp. Downsample" -> [w3055]
      tunnel: [w3058] -> w2549
      tunnel: w2381 -> [w3054]
      n1765 = call "integrate 1D array interval - double.vi"("Ave N"=w3055, "Array In"=w3057) -> ("Array Out"=w3056:dbl[])  [unwired: 1 out]
      n1766 = Multiply(x=w3065, y=w3055) -> (x*y=w3058:dbl)
      n1767 = Divide(x=w3056, y=w3062) -> (x/y=w3063:dbl[])
      n1768 = Bundle By Name("t0"=w3054, "Y"=w3063, "dt"=w3058) -> (w3064:waveform(dbl))  [unwired: 1 out]
      n1769 = Set Waveform Attribute(5:w3059, 6:w3060, 7:w3064) -> (3:w3061:waveform(dbl))  [unwired: 1 in, 2 out]
    }
    "APD Display Period (s)" <- w2549
    n1770 = Reciprocal(x=w2549) -> (1/x=→"APD Display Freq. (Hz)":dbl)
    n1771 = local read "Display Period (s)"() -> (w2439:dbl)
    n1772 = Increment(x=w2534) -> (x+1=w2535:dbl)
    n1773 = Index Array(array=w2334, index=0) -> (element=w2332:waveform(dbl))
    n1774 = To Double Precision Float(number=w2450) -> (double precision float=w2449:dbl[])
    n1775 = feedback #2(w2535) -> (w2538:dbl)
    n1776 = Select(t=0, s=w2525, f=w2538) -> (s? t:f=w2531:dbl)
    n1777 = Array Size(array=w2449) -> (size(s)=w2537:i32)
    n1778 = Add(x=w2537, y=w2531) -> (x+y=w2532:dbl)
    n1779 = Unbundle By Name(w2332) -> ("Y"=w2330:dbl[])
    n1780 = feedback #3(w2450) -> (w2521:u32[])
    n1781 = Build Array (concatenate)(w2521, w2450) -> (w2518:u32[])
    n1782 = feedback #4(w2395) -> (w2414:u32[])
    n1783 = Divide(x="Bead Sep. Int. Time (s)", y=w2439) -> (x/y=w2328:dbl)
    n1784 = Build Array (concatenate)(w2414, w2395) -> (w2413:u32[])
    n1785 = Greater?(x=w2532, y=w2534) -> (0:w2533:bool)
    n1786 = feedback #5(w2330) -> (w2331:dbl[])
    n1787 = Build Array (concatenate)(w2330, w2331) -> (w2329:dbl[])
    n1788 = Select(t=w2531, s=w2533, f=w2532) -> (s? t:f=w2530:dbl)
    n1789 = feedback-in #2(w2530) -> ()
    n1790 = Array Size(array=w2518) -> (size(s)=w2515:i32)
    n1791 = Array Size(array=w2450) -> (size(s)=w2517:i32)
    n1792 = local read "MCL Scanning"() -> (w2528:bool)
    n1793 = local read "APD Integration Time (s)"() -> (w2422:dbl)
    n1794 = Build Array (concatenate)(w2415, w2554) -> (w2417:waveform(dbl)[])
    "All Signals" <- w2417
    n1795 = Split 1D Array(array=w2329, index=w2328) -> (first subarray=w2322:dbl[])  [unwired: 1 out]
    n1796 = feedback-in #5(w2322) -> ()
    n1797 = Multiply(x=w2517, y="APD Ave N") -> (x*y=w2516:dbl)
    n1798 = Greater?(x=w2515, y=w2516) -> (0:w2519:bool)
    n1799 = Not(x=w2533) -> (.not. x?=w2527:bool)
    n1800 = To Double Precision Float(number=w2395) -> (double precision float=w2394:dbl[])
    n1801 = call-poly <vilib>:"Mean.vi"("X"=w2322) -> ("mean"=w2321:dbl)  [unwired: 1 out]
    "Mean T1 Position (nm)" <- w2321
    n1802 = Subtract(x=w2322, y=w2321) -> (x-y=w2327:dbl[])
    n1803 = Square(x=w2327) -> (x^2=w2326:dbl[])
    n1804 = And(x=w2527, y=w2528) -> (x .and. y?=w2529:bool)
    n1805 = call-poly <vilib>:"Mean.vi"("X"=w2326) -> ("mean"=w2325:dbl)  [unwired: 1 out]
    n1806 = case shown="True" w2519 {
      tunnel: w2518 -> [w2838 w2845]
      tunnel: [w2838 w2843] -> w2466
      tunnel: w2516 -> [_ w2840]
      tunnel: w2515 -> [_ w2844]
      tunnel: w2413 -> [w2837 w2842]
      tunnel: [w2837 w2839] -> w2410
      frame False {
      }
      frame True {
        n1807 = Subtract(x=w2844, y=w2840) -> (x-y=w2841:dbl)
        n1808 = Array Subset(array=w2845, index=w2841, length=w2840) -> (w2843:u32[])
        n1809 = Array Subset(array=w2842, index=w2841, length=w2840) -> (w2839:u32[])
      }
    }
    n1810 = feedback-in #3(w2466) -> ()
    n1811 = feedback-in #4(w2410) -> ()
    n1812 = Or(x=w2529, y=w2525) -> (x .or. y?=w2526:bool)
    n1813 = Square Root(x=w2325) -> (sqrt(x)=w2324:dbl)
    n1814 = Equal?(x="Tab Control Display", y=T36."High Res Display") -> (x = y?=w2456:bool)
    n1815 = Multiply(x="APD Disp. Scale", y=w2415) -> (x*y=w2424:waveform(dbl)[])
    n1816 = Multiply(x="APD Disp. Downsample", y=w2422) -> (x*y=w2420:dbl)
    n1817 = Multiply(x=10.0, y=w2324) -> (x*y=→"Trap 1 Position RMS (A)":dbl)
    n1818 = Divide(x=w2424, y=w2420) -> (x/y=w2392:waveform(dbl)[])
    n1819 = Index Array(array=w2392, index=0) -> (element=w2402:waveform(dbl))
    n1820 = case "For computing FFTs for display" shown="True" "Compute FFT" {
      tunnel: w2419 -> [_ w3522]
      frame False {
      }
      frame True {
        n1821 = Build Array("FFT 1 Choice 1", "FFT 1 Choice 2", "FFT 2 Choice 1", "FFT 2 Choice 2") -> (w3515:u16[])
        n1822 = Array Size(array=w3522) -> (size(s)=w3521:i32)
        n1823 = feedback-in #6(w3515) -> ()
        n1824 = feedback #6(u16[] [100, 100, 100, 100]) -> (w3516:u16[])
        n1825 = feedback-in #7("# Spectra to Ave.") -> ()
        n1826 = feedback #7("# Spectra to Ave.") -> (w3513:dbl)
        n1827 = Not Equal?(x="# Spectra to Ave.", y=w3513) -> (x != y?=w3512:bool)
        n1828 = Not Equal?(x=w3515, y=w3516) -> (x != y?=w3514:bool)
        n1829 = feedback #8(1.0) -> (w3499:dbl)
        n1830 = Compound Arithmetic op=OR("Reset FFT", w3514, w3512) -> (w3497:bool)
        n1831 = Select(t=1.0, s=w3497, f=w3499) -> (s? t:f=w3501:dbl)
        n1832 = Greater?(x=w3501, y="# Spectra to Ave.") -> (0:w3520:bool)
        n1833 = Increment(x=w3501) -> (x+1=w3500:dbl)
        n1834 = feedback-in #8(w3500) -> ()
        n1835 = local read "DMA Update Period (s)"() -> (w3495:dbl)
        n1836 = Multiply(x="# Spectra to Ave.", y=w3495) -> (x*y=→"Ave. Time (s)":dbl)
        n1837 = Build Array(cluster{"f0":dbl, "df":dbl, "magnitude":dbl[]} {"f0"=0.0, "df"=0.0, "magnitude"=[]} ("PSD")) -> (w3504:cluster{"f0":dbl, "df":dbl, "magnitude":dbl[]}[])
        n1838 = Build Array(w3504, w3504, w3504, w3504) -> (w3506:T47)
        n1839 = feedback #9(w3506) -> (w3511:T47)
        n1840 = for {
          N: 4 -> [_]
          tunnel: w3515 -> [w3544] mode=indexing
          tunnel: w3522 -> [w3545]
          tunnel: w3521 -> [w3547]
          tunnel: w3497 -> [w3540]
          tunnel: w3520 -> [w3539]
          tunnel: "# Spectra to Ave." -> [w3538]
          tunnel: [w3537] -> w3510 mode=indexing
          tunnel: w3511 -> [w3542] mode=indexing
          tunnel: [w3541] -> w3498 mode=indexing
          tunnel: w3501 -> [w3536]
          n1841 = Less?(x=w3544, y=w3547) -> (x < y?=w3546:bool)
          n1842 = Index Array(array=w3545, index=w3544) -> (element=w3543:waveform(dbl))
          n1843 = case shown="True" w3546 {
            tunnel: w3543 -> [_ w3564]
            tunnel: w3542 -> [w3549 w3562]
            tunnel: [w3549 w3550] -> w3541
            tunnel: w3540 -> [_ w3561]
            tunnel: w3539 -> [_ w3554]
            tunnel: w3538 -> [_ w3553]
            tunnel: [cluster{"f0":dbl, "df":dbl, "magnitude":dbl[]} {"f0"=0.0, "df"=0.0, "magnitude"=[]} ("PSD") w3555] -> w3537
            tunnel: w3536 -> [_ w3552]
            frame False {
            }
            frame True {
              n1844 = call <vilib>:"Std Deviation and Variance.vi"("X"=w3564) -> ("mean"=w3565:dbl)  [unwired: 1 in, 2 out]
              n1845 = Subtract(x=w3564, y=w3565) -> (x-y=w3563:waveform(dbl))
              n1846 = xnode "Spectral Measurements"("Signals"=w3563) -> ("PSD"=w3557:cluster{"f0":dbl, "df":dbl, "magnitude":dbl[]})  [unwired: 1 in, 1 out]
              n1847 = case shown="False" w3561 {
                tunnel: w3562 -> [w3574 _]
                tunnel: [w3570 w3579] -> w3550
                tunnel: w3557 -> [w3573 w3580]
                tunnel: w3554 -> [w3572 _]
                frame False {
                  n1848 = Build Array (concatenate)(w3574, w3573) -> (w3571:cluster{"f0":dbl, "df":dbl, "magnitude":dbl[]}[])
                  n1849 = case shown="True" w3572 {
                    tunnel: w3571 -> [w3575 w3578]
                    tunnel: [w3575 w3576] -> w3570
                    frame False {
                    }
                    frame True {
                      n1850 = Delete From Array(array=w3578, index=0) -> (array with subset deleted=w3576:cluster{"f0":dbl, "df":dbl, "magnitude":dbl[]}[])  [unwired: 1 in, 1 out]
                    }
                  }
                }
                frame True {
                  n1851 = Build Array(w3580) -> (w3579:cluster{"f0":dbl, "df":dbl, "magnitude":dbl[]}[])
                }
